vi "Auton File Loop.vi"   [LabVIEW 2013]
uses:
  Robot Global Data.vi
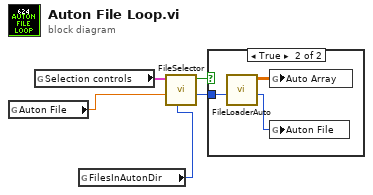
[diagram p0: block diagram]
diagram:
  n1 = global read "Robot Global Data.vi" "Auton File"() -> (w1:dbl)
  n2 = global read "Robot Global Data.vi" "Selection controls"() -> (w4:cluster{"Up":bool, "Down":bool})
  n3 = global read "Robot Global Data.vi" "FilesInAutonDir"() -> (w3:i32)
  n4 = call "FileSelector.vi"("array size"=w3, "index in"=w1, "Selection Controls"=w4) -> ("index out"=w2:i32, "isChanged"=w5:bool)  [unwired: 7 in]
  n5 = case shown="True" w5 {
    tunnel: w2 -> [_ w8]
    frame False {
    }
    frame True {
      n6 = call "FileLoaderAuto.vi"("index"=w8) -> ("coerced index"=w6:i32, "Auto Array"=w7:dbl[][])  [unwired: 9 in]
      n7 = global write "Robot Global Data.vi" "Auto Array"(w7) -> ()
      n8 = global write "Robot Global Data.vi" "Auton File"(w6) -> ()
    }
  }
